vi "Untitled 1 (SubVI).vi"(11 "data in":dbl[](array[numeric])) -> (3 "data out":dbl[](array[numeric]) format="%0.2f")   [LabVIEW 2017]
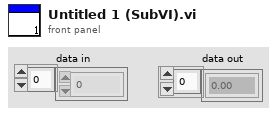
[diagram p1: front panel]
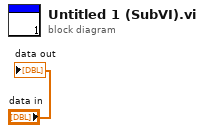
[diagram p0: block diagram]
diagram:
  "data out" <- "data in"
